vi "New Color.vi"(0 "Current Colors":u32[](array[colorbox])=[16711680], 11 "error in (no error)":errorcluster) -> (4 "Colors Out":u32[](array[colorbox]), 15 "error out":errorcluster)   [LabVIEW 2012, in "Picture Box Tools.lvlib"]
doc: "This VI generates a new color that is equadistant in hue variation from colors present in an array of colors. Use this VI to populate programmatically generated colors for a list or graph or display without repeating colors.\n\nSee HSLToolsAdvancedExample.vi in the NI Example Finder for more information."
uses:
  Picture Box Tools.lvlib
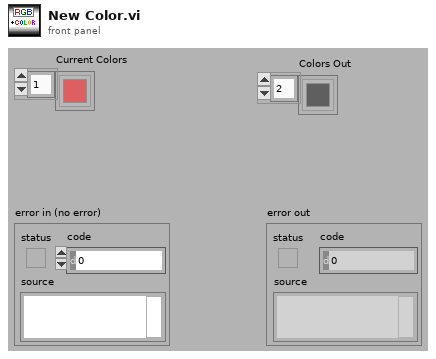
[diagram p1: front panel]
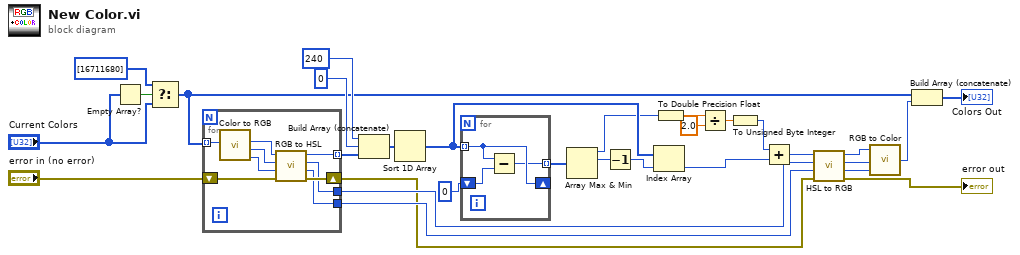
[diagram p0: block diagram]
diagram:
  n1 = Empty Array?(array="Current Colors") -> (empty?=w4:bool)
  n2 = Select(t=u32[] [16711680] ("Current Colors"), s=w4, f="Current Colors") -> (s? t:f=w1:u32[])
  n3 = for {
    tunnel: w1 -> [w35] mode=indexing
    shift-right: [w34] -> w12
    shift-left: "error in (no error)" -> [w36]
    tunnel: [w33] -> w8 mode=indexing
    tunnel: [w32] -> w14
    tunnel: [w31] -> w13
    n4 = call <vilib>:"Color to RGB.vi"("Color"=w35) -> ("R"=w39:u8, "G"=w38:u8, "B"=w37:u8)  [unwired: 1 out]
    n5 = call <vilib>:"RGB to HSL.vi"("Error In"=w36, "Blue"=w37, "Green"=w38, "Red"=w39) -> ("Error Out"=w34:errorcluster, "Lum"=w31:u8, "Sat"=w32:u8, "Hue"=w33:u8)  [unwired: 4 out]
  }
  n6 = Build Array (concatenate)(u8 240 ("Hue"), u8 0 ("Hue"), w8) -> (w5:u8[])
  n7 = Sort 1D Array(array=w5) -> (sorted array=w25:u8[])
  n8 = for {
    tunnel: w25 -> [w42] mode=indexing
    shift-right: [w42] -> _
    shift-left: u8 0 ("Hue") -> [w41]
    tunnel: [w40] -> w28 mode=indexing
    n9 = Subtract(x=w42, y=w41) -> (x-y=w40:u8)
  }
  n10 = Array Max & Min(array=w28) -> (max value=w24:u8, max index (indices)=w27:i32)  [unwired: 2 out]
  n11 = Decrement(x=w27) -> (x-1=w26:i32)
  n12 = Index Array(array=w25, index=w26) -> (element=w20:u8)
  n13 = To Double Precision Float(number=w24) -> (double precision float=w23:dbl)
  n14 = Divide(x=w23, y=2.0) -> (x/y=w21:dbl)
  n15 = To Unsigned Byte Integer(number=w21) -> (unsigned 8bit integer=w19:u8)
  n16 = Add(x=w19, y=w20) -> (x+y=w15:u8)
  n17 = call <vilib>:"HSL to RGB.vi"("Error In"=w12, "Lum"=w13, "Sat"=w14, "Hue"=w15) -> ("Error Out"=→"error out":errorcluster, "Blue"=w16:u8, "Green"=w17:u8, "Red"=w18:u8)  [unwired: 4 out]
  n18 = call <vilib>:"RGB to Color.vi"("B"=w16, "G"=w17, "R"=w18) -> ("Color"=w10:u32)
  n19 = Build Array (concatenate)(w1, w10) -> (→"Colors Out":u32[])
